vi "Close.vi"(8 "error in (no error)":errorcluster, 11 "BaseDriver in":refnum<class "BaseDriver.lvclass">) -> (0 "error out":errorcluster, 3 "BaseDriver out":refnum<class "BaseDriver.lvclass">)   [LabVIEW 2013, in "BaseDriver.lvclass"]
doc: "Closes all open references and reserved resources for the driver"
uses:
  BaseDriver.lvclass
  BaseDriver.lvclass/BaseDriver.ctl
  Reader/BaseReader/BaseReader.lvclass
  Responder/BaseResponder/BaseResponder.lvclass
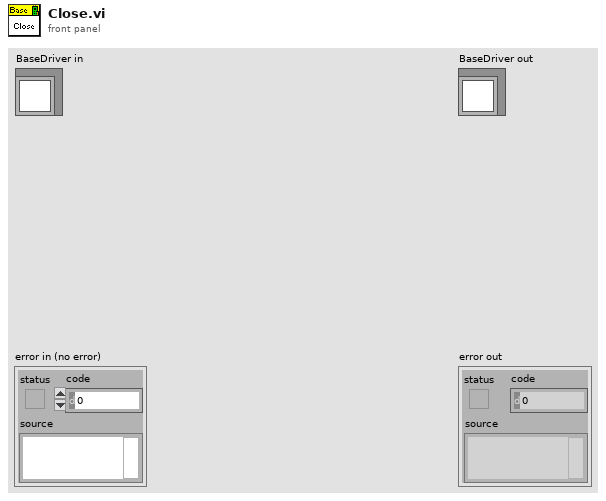
[diagram p1: front panel]
types:
  T1 = typedef "message_queue.ctl" = refnum<queue>
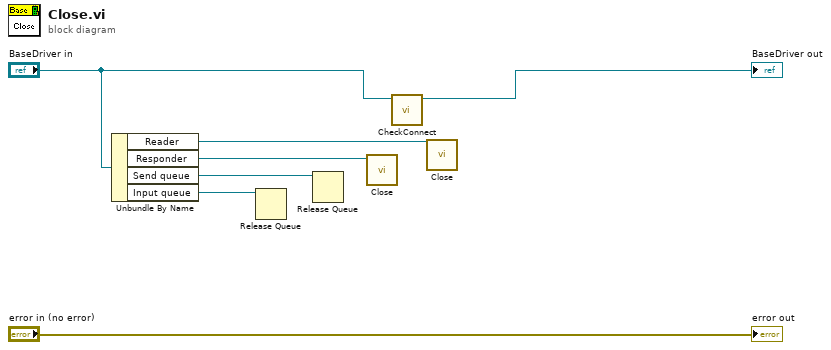
[diagram p0: block diagram]
diagram:
  n1 = Unbundle By Name("BaseDriver in") -> ("Reader"=w4:refnum<class "BaseReader.lvclass">, "Responder"=w3:refnum<class "BaseResponder.lvclass">, "Send queue"=w5:T1, "Input queue"=w6:T1)
  n2 = Release Queue(queue=w6) -> ()  [unwired: 2 in, 3 out]
  n3 = Release Queue(queue=w5) -> ()  [unwired: 2 in, 3 out]
  n4 = call-dynamic "Close.vi"("BaseResponder in"=w3) -> ()  [unwired: 9 in, 2 out]
  n5 = call "CheckConnect.vi"("BaseDriver in"="BaseDriver in") -> ("BaseDriver out"=→"BaseDriver out":refnum<class "BaseDriver.lvclass">)  [unwired: 9 in, 1 out]
  n6 = call-dynamic "Close.vi"("BaseReader in"=w4) -> ()  [unwired: 9 in, 2 out]
  "error out" <- "error in (no error)"
